vi "PrettyPrint.vi"() -> ()   [LabVIEW 2015]
uses:
  <vilib>/xml/Load XML File.vi
  <vilib>/xml/Close Reference(Node).vi
  <vilib>/xml/NI_XML.lvlib
  <resource>/objmgr/DOMUserDefRef.rc
panel:
  in  "Output_File":path caption="OutputFile"
  out "XML":string
  in  "XML_File":path
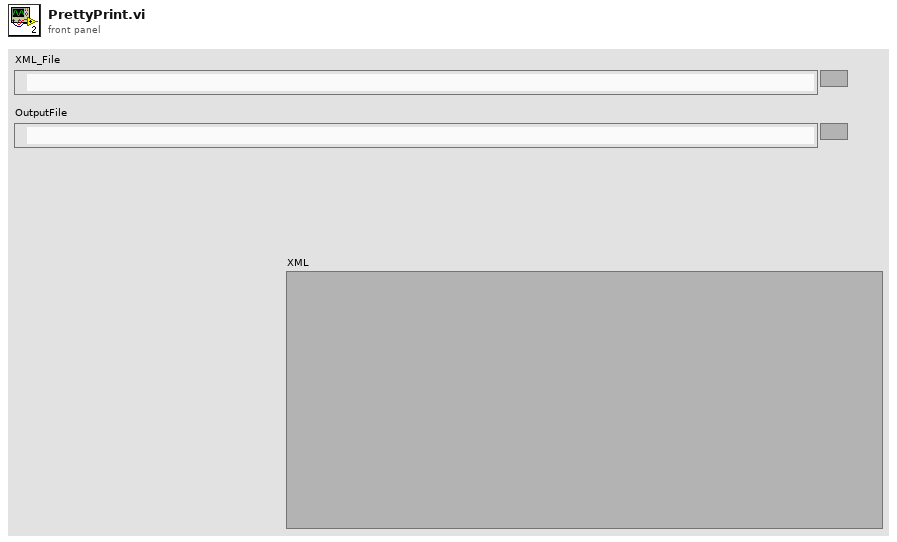
[diagram p1: front panel]
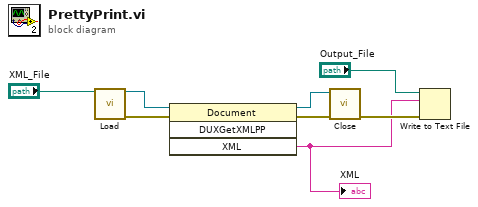
[diagram p0: block diagram]
diagram:
  n1 = call-poly <vilib>:"Load.vi"("path to XML document"="XML_File") -> ("DOM document out"=w7:refnum<k20>, "error out"=w8:errorcluster)  [unwired: 12 in, 1 out]
  n2 = invoke class="Document" method="DUXGetXMLPP"(reference=w7, error in=w8) -> (reference out=w4:refnum<k20>, error out=w5:errorcluster, "XML"=w2:string)  [unwired: 2 in, 1 out]
  "XML" <- w2
  n3 = call-poly <vilib>:"Close.vi"("error in (no error)"=w5, "node"=w4) -> ("error out"=w3:errorcluster)  [unwired: 7 in]
  n4 = Write to Text File(file (use dialog)="Output_File", text=w2, error in=w3) -> ()  [unwired: 1 in, 3 out]
